vi "WordValidation.vi"(8 "error in (no error)":errorcluster, 10 "Word":string, 11 "Controller in":refnum<class "Controller.lvclass">) -> (0 "error out":errorcluster, 2 "Valid?":bool, 3 "Controller out":refnum<class "Controller.lvclass">)   [LabVIEW 2024, in "GUI.lvlib" / "Controller.lvclass"]
uses:
  Controller.lvclass
  Controller.lvclass/Controller.ctl
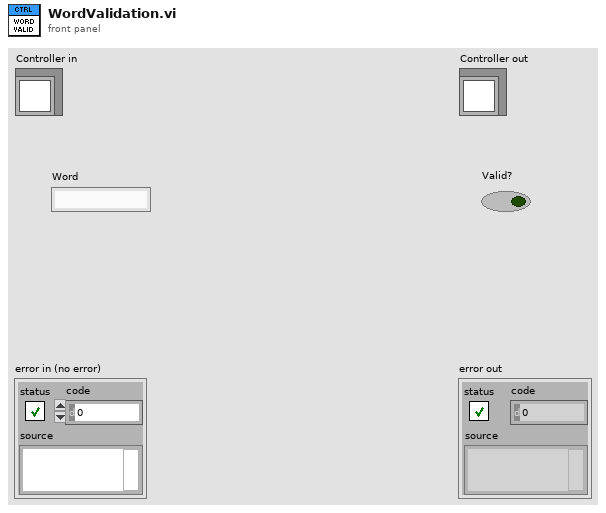
[diagram p1: front panel]
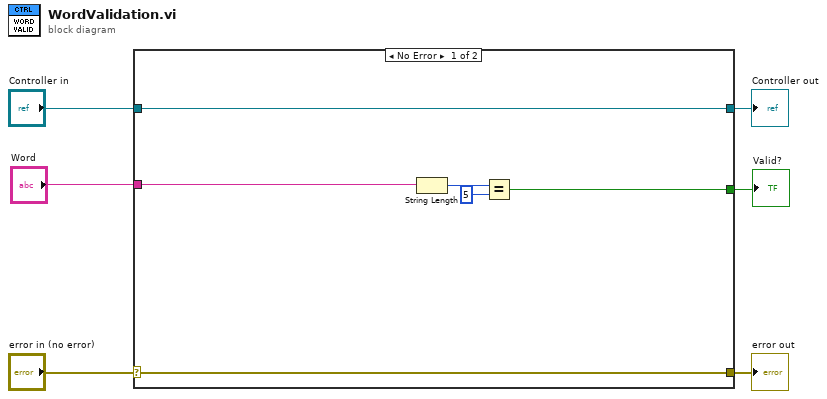
[diagram p0: block diagram]
diagram:
  n1 = case shown="No Error" "error in (no error)" {
    selector: "error in (no error)" -> [w11 w14]
    tunnel: [w11 w14] -> w5
    tunnel: [w12 w13] -> w3
    tunnel: "Controller in" -> [w12 w13]
    tunnel: "Word" -> [w10 _]
    tunnel: [w7 _] -> w1
    frame No Error {
      n2 = String Length(string=w10) -> (length=w9:i32)
      n3 = Equal?(x=w9, y=5) -> (x = y?=w7:bool)
    }
    frame Error {
    }
  }
  "error out" <- w5
  "Controller out" <- w3
  "Valid?" <- w1
